vi "a1.vi"() -> ()   [LabVIEW 2010]
panel:
  out "XY Graph":cluster{dbl[], dbl[]}[](graph)
  out "subarray 3":dbl[](array[numeric])
  out "subarray 2":dbl[](array[numeric])
  out "subarray":dbl[](array[numeric])
  in  "file path":path=path "C:/data/RUS/Experiment/ProbeTest/Probe8/SrKIr016/Sweep me baby 1/October_2011/102011/239.87300K_1250_2500_001_102011.dat"
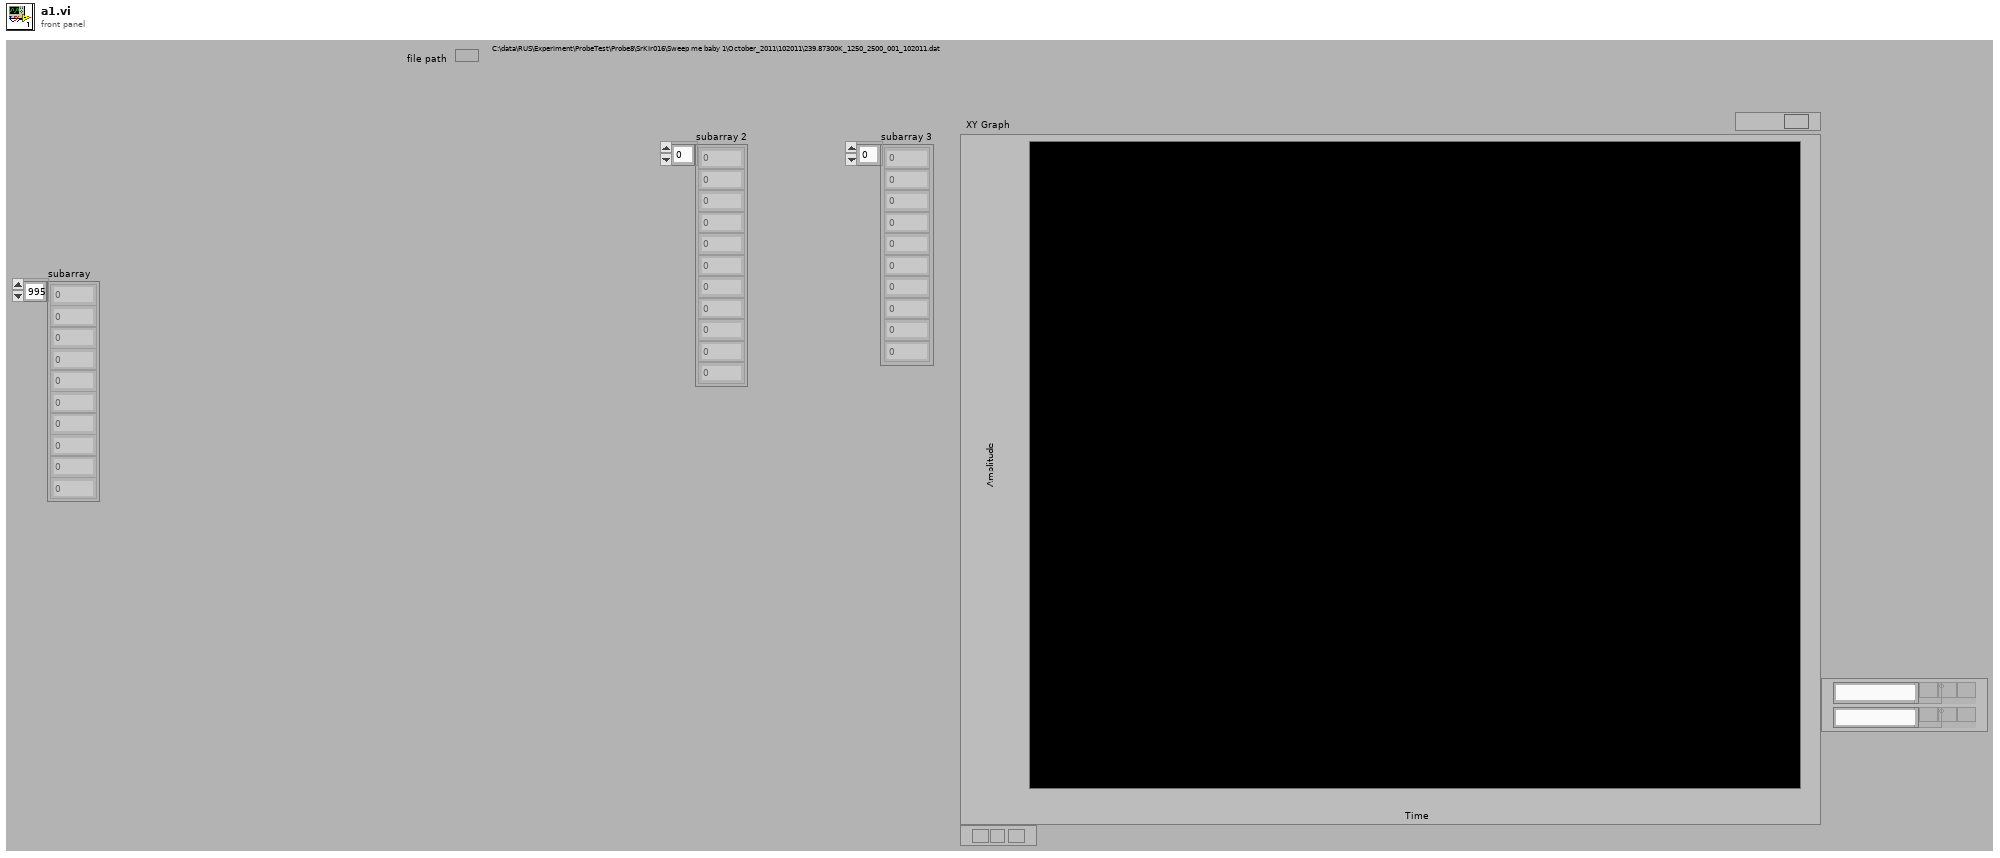
[diagram p1: front panel]
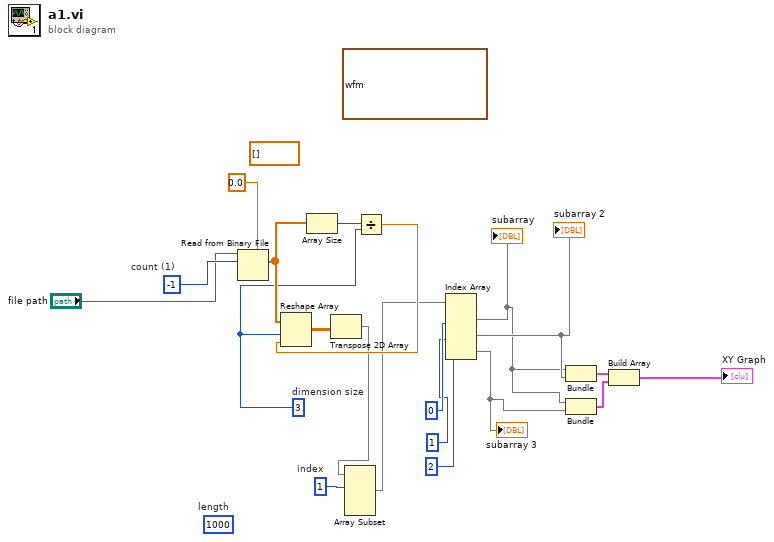
[diagram p0: block diagram]
diagram:
  (unwired) waveform(dbl) {"t0"=timestamp(0 s since 1904-01-01), "dt"=1.0, "Y"=[]} ("Waveform")
  (unwired) 1000  # length
  w6 = 1  # index
  w16 = 3  # dimension size
  w20 = -1  # count (1)
  (unwired) dbl[] []
  n1 = Read from Binary File(5:0.0, 10:w20, 11:"file path") -> (2:w18:dbl[])  [unwired: 3 in, 3 out]
  n2 = Array Size(array=w18) -> (size(s)=w17:i32)
  n3 = Divide(x=w17, y=w16) -> (x/y=w15:dbl)
  n4 = Reshape Array(w18, w16, w15) -> (w19:dbl[][])
  n5 = Transpose 2D Array(2D array=w19) -> (transposed array=w5:dbl[][])
  n6 = Array Subset(array=w5, index (row)=w6) -> (w4:dbl[][])  [unwired: 3 in]
  n7 = Index Array(array=w4, index (col) #1=0 ("disabled index (col)"), index (col) #2=1 ("disabled index (col)"), index (col) #3=2 ("disabled index (col)")) -> (element #1=w8:dbl[], element #2=w9:dbl[], element #3=w7:dbl[])  [unwired: 3 in]
  "subarray" <- w8
  "subarray 2" <- w9
  "subarray 3" <- w7
  n8 = Bundle(w8, w9) -> (w10:cluster{dbl[], dbl[]})  [unwired: 1 in]
  n9 = Bundle(w8, w7) -> (w3:cluster{dbl[], dbl[]})  [unwired: 1 in]
  n10 = Build Array(w10, w3) -> (→"XY Graph":cluster{dbl[], dbl[]}[])
